vi "InRanges__slk_mt.vi"(7 "segments in":refnum<class "Segment__slk_mt.lvclass">[](array[class]), 8 "error in (no error)":errorcluster, 10 "point":cluster{"x":i32, "y":i32}, 11 "view in":refnum<class "View__slk_mt.lvclass">) -> (0 "error out":errorcluster, 2 "range index":u16, 3 "in ranges?":bool)   [LabVIEW 2012, in "Lazyboots Menu Tool.lvlib"]
doc: "Check if the point is in ranges."
uses:
  Library/Lazyboots Menu Tool.lvlib
  Class/View/View__slk_mt.lvclass
  Class/Segment/Segment__slk_mt.lvclass
panel:
  # "InRanges__slk_mt.vi\nCheck if the point is in ranges.\n\nNOTICE -- YOU MUST LEAVE THIS NOTICE IN PLACE.\n\nCopyright (c) 2011, LIANG LIU Shawn.Liu.cn@gmail.com\nAll rights reserved.\n\nRedistribution and use in source and binary forms, with or without modification, are permitted provided that the following conditions are met:\n-Redistributions of source code must retain the above copyright notice, this list of conditions and the following disclaimer.\n-Redistributions in binary form must reproduce the above copyright notice, this list of conditions and the following disclaimer in the documentation and/or other materials provided with the distribution.\n-Neither the name of the eLp nor the names of its contributors may be used to endorse or promote products derived from this software without specific prior written permission.\n\nTHIS SOFTWARE IS PROVIDED BY THE COPYRIGHT HOLDERS AND CONTRIBUTORS \"AS IS\" AND ANY EXPRESS OR IMPLIED WARRANTIES, INCLUDING, BUT NOT LIMITED TO, THE IMPLIED WARRANTIES OF MERCHANTABILITY AND FITNESS FOR A PARTICULAR PURPOSE ARE DISCLAIMED. IN NO EVENT SHALL THE COPYRIGHT HOLDER OR CONTRIBUTORS BE LIABLE FOR ANY DIRECT, INDIRECT, INCIDENTAL, SPECIAL, EXEMPLARY, OR CONSEQUENTIAL DAMAGES (INCLUDING, BUT NOT LIMITED TO, PROCUREMENT OF SUBSTITUTE GOODS OR SERVICES; LOSS OF USE, DATA, OR PROFITS; OR BUSINESS INTERRUPTION) HOWEVER CAUSED AND ON ANY THEORY OF LIABILITY, WHETHER IN CONTRACT, STRICT LIABILITY, OR TORT (INCLUDING NEGLIGENCE OR OTHERWISE) ARISING IN ANY WAY OUT OF THE USE OF THIS SOFTWARE, EVEN IF ADVISED OF THE POSSIBILITY OF SUCH DAMAGE."
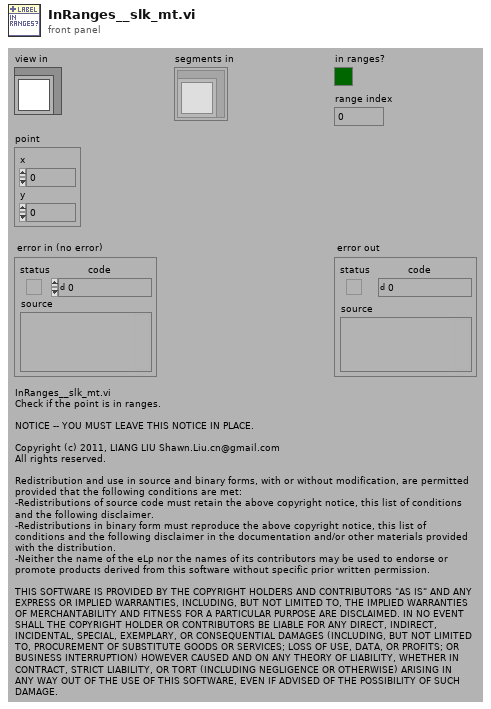
[diagram p1: front panel]
types:
  T1 = cluster{"left":sgl, "top":sgl, "right":sgl, "bottom":sgl}
  T2 = cluster{"left":i16, "top":i16, "right":i16, "bottom":i16}
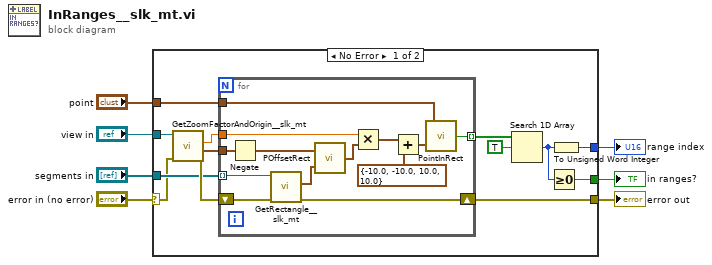
[diagram p0: block diagram]
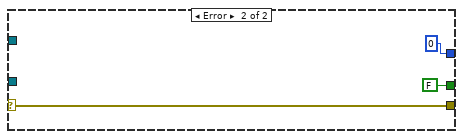
[diagram p2: hidden frame]
diagram:
  n1 = case shown="No Error" "error in (no error)" {
    selector: "error in (no error)" -> [w10 w36]
    tunnel: "view in" -> [w15 _]
    tunnel: [w14 u16 0] -> w6
    tunnel: "segments in" -> [w13 _]
    tunnel: [w11 FALSE] -> w4
    tunnel: [w9 w36] -> w2
    tunnel: "point" -> [w8 _]
    frame No Error {
      n2 = call "GetZoomFactorAndOrigin__slk_mt.vi"("error in (no error)"=w10, "view in"=w15) -> ("error out"=w17:errorcluster, "origin"=w18:cluster{"Horizontal":i16, "Vertical":i16}, "zoom factor"=w19:sgl)  [unwired: 6 in, 1 out]
      n3 = for {
        tunnel: w19 -> [w33]
        tunnel: w18 -> [w29]
        tunnel: [w32] -> w20 mode=indexing
        shift-right: [w23] -> w9
        shift-left: w17 -> [w25]
        tunnel: w13 -> [w22] mode=indexing
        tunnel: w8 -> [w21]
        n4 = Negate(x=w29) -> (-x=w26:cluster{"Horizontal":i16, "Vertical":i16})
        n5 = call "GetRectangle__slk_mt.vi"("error in (no error)"=w25, "segment in"=w22) -> ("error out"=w23:errorcluster, "rectangle"=w28:T2)  [unwired: 7 in, 1 out]
        n6 = call <vilib>:"POffsetRect.vi"("rect"=w28, "point"=w26) -> ("offset rect"=w27:T2)
        n7 = Multiply(x=w33, y=w27) -> (x*y=w31:T1)
        n8 = Add(x=w31, y=T1 {"left"=-10.0, "top"=-10.0, "right"=10.0, "bottom"=10.0} ("expand size")) -> (x+y=w30:T1)
        n9 = call <vilib>:"PointInRect.vi"("rect"=w30, "point"=w21) -> ("pt in rect"=w32:bool)
      }
      n10 = Search 1D Array(1D array=w20, element=TRUE) -> (index of element=w12:i32)  [unwired: 1 in]
      n11 = Greater Or Equal To 0?(x=w12) -> (x >= 0?=w11:bool)
      n12 = To Unsigned Word Integer(number=w12) -> (unsigned 16bit integer=w14:u16)
    }
    frame Error {
    }
  }
  "range index" <- w6
  "in ranges?" <- w4
  "error out" <- w2
